vi "Set Instr CFG.vi"(8 "Error In":errorcluster, 10 "Instr Ident":string, 11 "object in":refnum<class "Configuration UI Actor.lvclass">) -> (0 "Error Out":errorcluster, 3 "object out":refnum<class "Configuration UI Actor.lvclass">)   [LabVIEW 2023, in "Configuration UI Actor.lvlib" / "Configuration UI Actor.lvclass"]
uses:
  Configuration UI Actor.lvclass
  Configuration UI Actor.lvclass/Configuration UI Actor.ctl
  <vilib>/JDP Science/JSONtext/JSONtext.lvlib
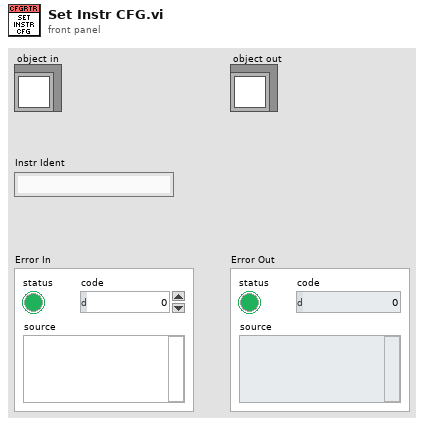
[diagram p1: front panel]
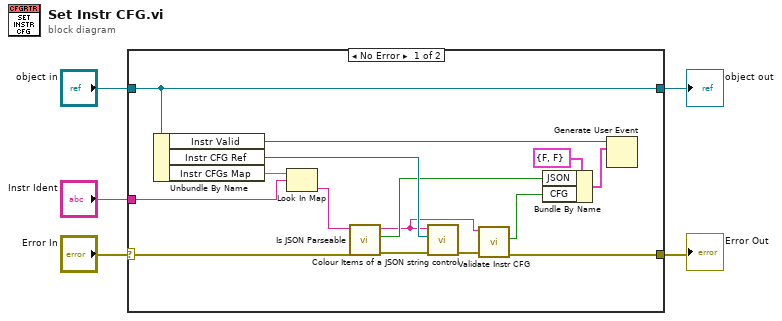
[diagram p0: block diagram]
diagram:
  n1 = case shown="No Error" "Error In" {
    selector: "Error In" -> [w17 w22]
    tunnel: [w6 w22] -> w4
    tunnel: [w20 w21] -> w2
    tunnel: "object in" -> [w20 w21]
    tunnel: "Instr Ident" -> [w18 _]
    frame No Error {
      n2 = Unbundle By Name(w20) -> ("Instr Valid"=w13:refnum<user-event>, "Instr CFG Ref"=w14:refnum<vi>, "Instr CFGs Map"=w19:map{string, string})
      n3 = Look In Map(map=w19, key=w18) -> (value=w16:string)  [unwired: 1 in, 1 out]
      n4 = call "Is JSON Parseable.vi"("error in (no error)"=w17, "<JSON>"=w16) -> ("error out"=w15:errorcluster, "Valid?"=w10:bool, "Pretty <JSON>"=w8:string)  [unwired: 7 in]
      n5 = call <vilib>:"Colour Items of a JSON string control.vi"("error in (no error)"=w15, "String Control"=w14, "JSON"=w8) -> ("error out"=w9:errorcluster)  [unwired: 8 in]
      n6 = call "Validate Instr CFG.vi"("Error In"=w9, "<JSON>"=w8) -> ("Error Out"=w6:errorcluster, "Is Valid?"=w7:bool)  [unwired: 8 in]
      n7 = Bundle By Name(cluster=cluster{"JSON":bool, "CFG":bool} {"JSON"=FALSE, "CFG"=FALSE} ("Instr Valid"), "JSON"=w10, "CFG"=w7) -> (w12:cluster{"JSON":bool, "CFG":bool})
      n8 = Generate User Event(user event=w13, event data cluster=w12) -> ()  [unwired: 2 in, 2 out]
    }
    frame Error {
    }
  }
  "Error Out" <- w4
  "object out" <- w2
